vi "CalibProcess.vi"(6 "ROI Descriptor":T2 {"Contours"."Type" items=["No Selection", "Point", "Line", "Rectangle", "Oval", "Polygon", "Freehand Region", "Annulus", "Unused2", "Unused3", "Broken Line", "Freehand Line", "Rotated Rectangle"]}, 7 "Area Max":dbl, 8 "error in (no error)":errorcluster, 9 "Area Min":dbl, 10 "ROI":T3, 11 "Refnum in":T1) -> (0 "error out":errorcluster, 2 "Image Dst Out":T1, 3 "Refnum out":T1(plugin-control))   [LabVIEW 2019]
uses:
  <vilib>/vision/Image Controls.llb/IMAQ Image.ctl
  <vilib>/vision/NI_Vision_Development_Module.lvlib
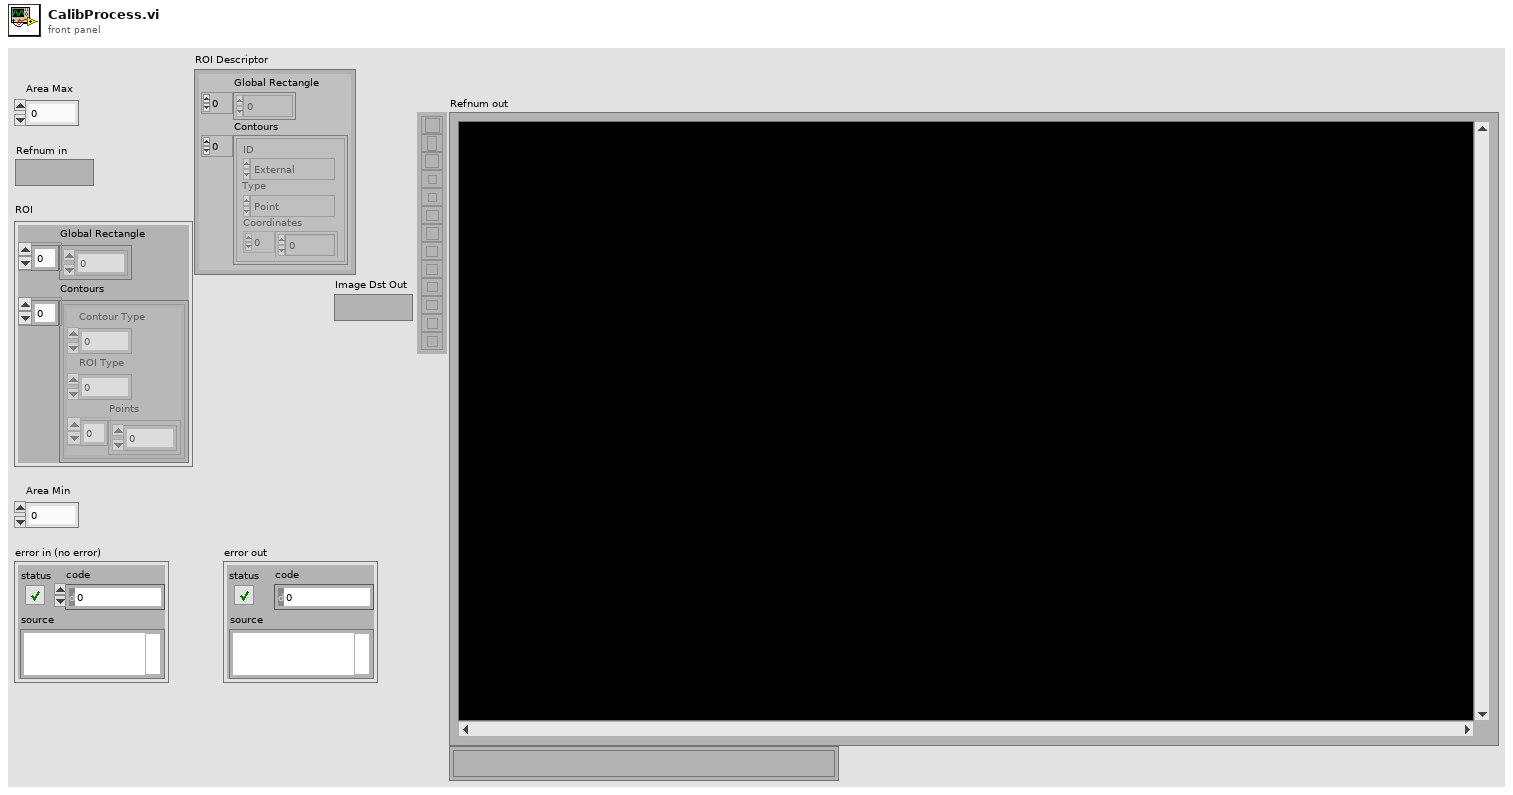
[diagram p1: front panel]
types:
  T1 = typedef "IMAQ Image.ctl" = refnum<image>
  T2 = typedef "ROI Descriptor" = cluster{"Global Rectangle":i32[], "Contours":cluster{"ID":enum32{"External", "Internal"}, "Type":u32, "Coordinates":i32[]}[]}
  T3 = cluster{"Global Rectangle":i32[], "Contours":cluster{"Contour Type":u32, "ROI Type":u32, "Points":i32[]}[]}
  T4 = typedef "Particle Parameters" = i32
  T5 = cluster{"Measurement Parameter":T4, "Range Lower Value":dbl, "Range Upper Value":dbl, "Range":bool, "Measurement Type":bool}
  T6 = typedef "Image Type" = u32
  T7 = cluster{"Measurement Parameter":T4, "Range Lower Value":dbl, "Range Upper Value":dbl, "Range":bool, "Measurement Type":bool}[]
  T8 = cluster{"Area":dbl, "Number of Holes":dbl, "Bounding Rect":cluster{"Left":dbl, "Top":dbl, "Right":dbl, "Bottom":dbl}, "Center of Mass":cluster{"X":dbl, "Y":dbl}, "Orientation":dbl, "Dimensions":cluster{"Width":dbl, "Height":dbl}}[]
  T9 = cluster{"Left":dbl, "Top":dbl, "Right":dbl, "Bottom":dbl}
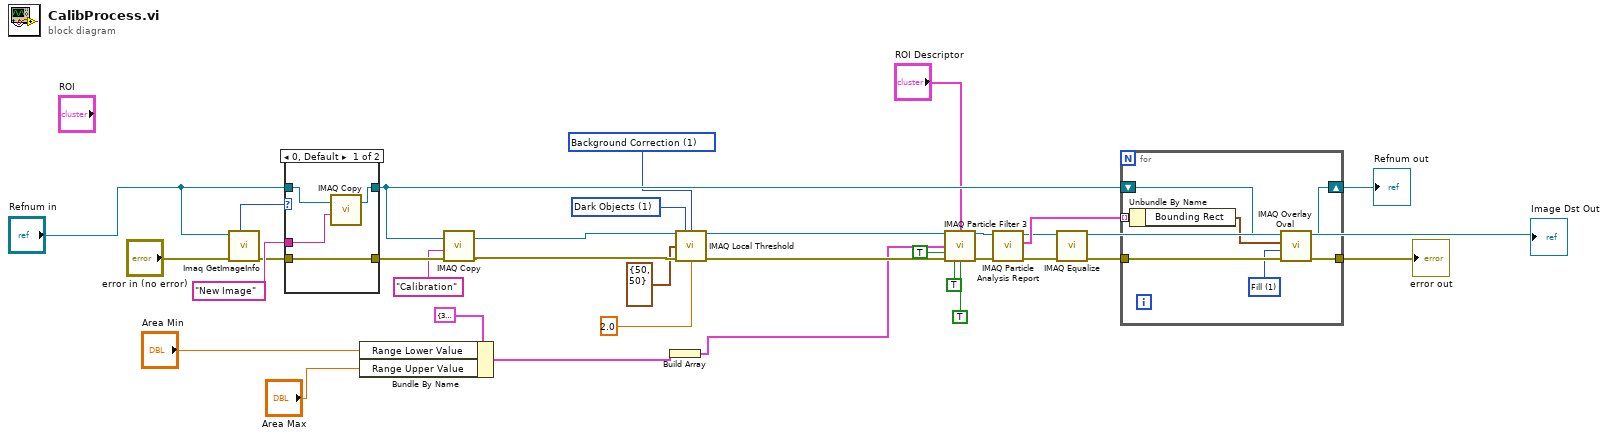
[diagram p0: block diagram]
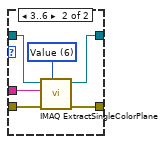
[diagram p2: hidden frame]
diagram:
  w16 = u32 1 items=["Niblack", "Background Correction"] ("Method (Niblack)")
  w17 = u32 1 items=["Bright Objects", "Dark Objects"] ("Look For (Bright Objects)")
  n1 = call "Imaq GetImageInfo"("error in (no error)"="error in (no error)", "Image"="Refnum in") -> ("error out"=w22:errorcluster, "Image Type"=w20:T6)  [unwired: 2 in, 6 out]
  n2 = case shown="0, Default" w20 {
    tunnel: "Refnum in" -> [w36 w44]
    tunnel: w22 -> [w38 w43]
    tunnel: [w37 w42] -> w27
    tunnel: [w38 w41] -> w24
    tunnel: "New Image" ("Image Name") -> [w35 w39]
    frame 0, Default {
      n3 = call "IMAQ Copy"("Image Dst"=w35, "Image Src"=w36) -> ("Image Dst Out"=w37:T1)  [unwired: 4 in, 1 out]
    }
    frame 3..6 {
      w40 = 6 items=["Red", "Green", "Blue", "Hue", "Saturation", "Luminance", "Value", "Intensity"] ("Color Plane")
      n4 = call "IMAQ ExtractSingleColorPlane"("Color Plane"=w40, "error in (no error)"=w43, "Image Dst"=w39, "Image Src"=w44) -> ("error out"=w41:errorcluster, "Image Dst Out"=w42:T1)  [unwired: 6 in]
    }
  }
  n5 = Bundle By Name(cluster=T5 {"Measurement Parameter"=35, "Range Lower Value"=0.0, "Range Upper Value"=500.0, "Range"=TRUE, "Measurement Type"=FALSE} ("Selection Value"), "Range Lower Value"="Area Min", "Range Upper Value"="Area Max") -> (w10:T5)
  n6 = call "IMAQ Copy"("error in (no error)"=w24, "Image Dst"="Calibration" ("Image Name"), "Image Src"=w27) -> ("error out"=w25:errorcluster, "Image Dst Out"=w26:T1)  [unwired: 3 in]
  n7 = Build Array(w10) -> (w3:T7)
  n8 = call "IMAQ Local Threshold"("Image Src"=w26, "Look For (Bright Objects)"=w17, "Method (Niblack)"=w16, "Window Size (32x32)"=cluster{"SizeX":i32, "SizeY":i32} {"SizeX"=50, "SizeY"=50}, "error in (no error)"=w25, "Replace Value (1)"=sgl 2.0) -> ("Image Dst Out"=w15:T1, "error out"=w14:errorcluster)  [unwired: 3 in, 5 out]
  n9 = call "IMAQ Particle Filter 3"("Image Src"=w15, "ROI Descriptor"="ROI Descriptor", "Selection Values"=w3, "Keep/Remove Particles (F)"=TRUE, "error in (no error)"=w14, "Reject Border? (F)"=TRUE, "Fill Holes? (F)"=TRUE) -> ("Image Dst Out"=w5:T1, "error out"=w6:errorcluster)  [unwired: 2 in, 5 out]
  n10 = call "IMAQ Particle Analysis Report"("error in (no error)"=w6, "Image"=w5) -> ("error out"=w29:errorcluster, "Particle Reports (Pixels)"=w33:T8, "Image Out (duplicate)"=w31:T1)  [unwired: 4 in, 3 out]
  n11 = call "IMAQ Equalize"("error in (no error)"=w29, "Image Src"=w31) -> ("error out"=w30:errorcluster, "Image Dst Out"=→"Image Dst Out":T1)  [unwired: 8 in]
  n12 = for {
    tunnel: w30 -> [w51]
    tunnel: [w50] -> w32
    tunnel: w33 -> [w49] mode=indexing
    shift-right: [w45] -> w28
    shift-left: w27 -> [w47]
    w46 = u32 1 items=["Frame", "Fill"] ("Drawing Mode (Frame)")
    n13 = Unbundle By Name(w49) -> ("Bounding Rect"=w48:T9)
    n14 = call "IMAQ Overlay Oval"("error in (no error)"=w51, "Drawing Mode (Frame)"=w46, "Bounding Rectangle"=w48, "Image"=w47) -> ("error out"=w50:errorcluster, "Image Out"=w45:T1)  [unwired: 6 in]
  }
  "error out" <- w32
  "Refnum out" <- w28
